vi "ErrorHandler.vi"(1 "BOOLEAN":i8) -> (0 "error out":errorcluster)   [LabVIEW 2014, in "Sixpack - Driver.lvlib"]
doc: "ACHTUNG: Bei rotatorischen Achsen sind bei MT_NULLLEFT = 0 nur negative, bei MT_NULLLEFT = 1 nur positive Werte definiert! Der Motor fährt von der aktuellen Position auf die Zielposition. Das Kommando wird nicht ausgeführt, wenn der Motor noch in der Rampenfahrt ist. Um die Zielposition für einen sich bewegenden Motor zu ändern, siehe Kapitel 3.6.3\n\nCMD $23\nMotorNr (0...5)\nTargetPosition"
uses:
  Sixpack - Driver.lvlib
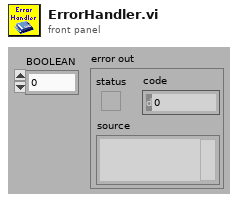
[diagram p1: front panel]
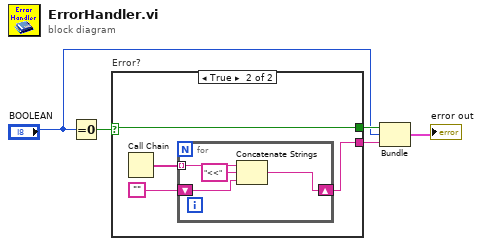
[diagram p0: block diagram]
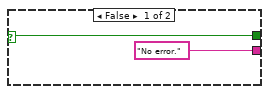
[diagram p2: hidden frame]
diagram:
  n1 = Equal To 0?(x="BOOLEAN") -> (x = 0?=w5:bool)
  n2 = case "Error?" shown="True" w5 {
    selector: w5 -> [w7 w11]
    tunnel: [w7 w11] -> w4
    tunnel: ["No error." w8] -> w1
    frame False {
    }
    frame True {
      n3 = Call Chain() -> (call chain=w10:string[])
      n4 = for {
        tunnel: w10 -> [w15] mode=indexing
        shift-right: [w12] -> w8
        shift-left: "" -> [w13]
        n5 = Concatenate Strings(w15, "<<" ("string"), w13) -> (w12:string)
      }
    }
  }
  n6 = Bundle(w4, "BOOLEAN"="BOOLEAN", w1) -> (→"error out":cluster{bool, "BOOLEAN":i8, string})  [unwired: 1 in]
